vi "GetSyncRefnums.vi"(8 "error in (no error)":errorcluster, 11 "ModuleAdmin":refnum<class "ModuleAdmin.lvclass">) -> (0 "error out":errorcluster, 1 "rndzv_ModuleSync":T1, 2 "rndzv_EventSync":T1, 3 "rndzv_StopSync":T1)   [LabVIEW 2018, in "ModuleAdmin.lvlib" / "ModuleAdmin.lvclass"]
uses:
  ModuleAdmin.lvclass
  ModuleAdmin.lvclass/ModuleAdmin.ctl
  Accessors/Read CloneRegRef.vi
  CloneRegistration/CloneRegistration.lvclass
panel:
  out "new StopSync":bool
  out "new EventSync":bool
  out "new ModuleSync":bool
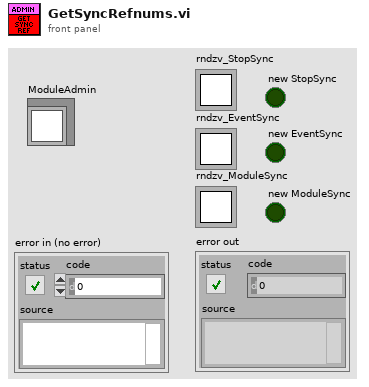
[diagram p1: front panel]
types:
  T1 = typedef "Rendezvous RefNum" = refnum<k1>
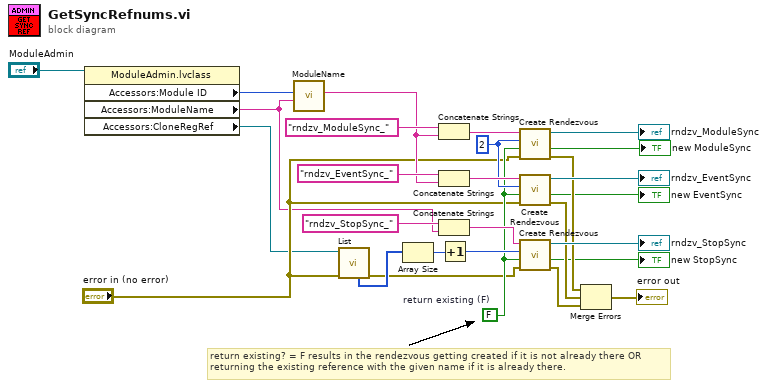
[diagram p0: block diagram]
diagram:
  w18 = 2 ("size (2)")
  w10 = FALSE  # return existing (F)
  # "return existing? = F results in the rendezvous getting created if it is not already there OR\nreturning the existing reference with the given name if it is already there."
  n1 = property class="ModuleAdmin.lvclass"(reference="ModuleAdmin") -> ("Accessors:Module ID"=w3:i32, "Accessors:ModuleName"=w1:string, "Accessors:CloneRegRef"=w2:refnum<data-value>)  [unwired: 1 in, 2 out]
  n2 = call "ModuleName.vi"("Name"=w1, "ModuleID"=w3) -> ("ModuleName"=w22:string)  [unwired: 9 in]
  n3 = call "List.vi"("error in (no error)"="error in (no error)", "CloneRegRef"=w2) -> ("error out"=w5:errorcluster, "Module IDs"=w28:i32[])  [unwired: 4 in, 4 out]
  n4 = Array Size(array=w28) -> (size(s)=w27:i32)
  n5 = Concatenate Strings("rndzv_ModuleSync_" ("string"), w22) -> (w21:string)
  n6 = Concatenate Strings("rndzv_EventSync_" ("string"), w22) -> (w20:string)
  n7 = Concatenate Strings("rndzv_StopSync_" ("string"), w1) -> (w19:string)
  n8 = Increment(x=w27) -> (x+1=w26:i32)
  n9 = call <vilib>:"Create Rendezvous.vi"("error in (no error)"="error in (no error)", "return existing (F)"=w10, "size (2)"=w18, "name (unnamed)"=w21) -> ("error out"=w13:errorcluster, "created new"=→"new ModuleSync":bool, "rendezvous"=→"rndzv_ModuleSync":T1)  [unwired: 1 in]
  n10 = call <vilib>:"Create Rendezvous.vi"("error in (no error)"="error in (no error)", "return existing (F)"=w10, "size (2)"=w18, "name (unnamed)"=w20) -> ("error out"=w14:errorcluster, "created new"=→"new EventSync":bool, "rendezvous"=→"rndzv_EventSync":T1)  [unwired: 1 in]
  n11 = call <vilib>:"Create Rendezvous.vi"("error in (no error)"=w5, "return existing (F)"=w10, "size (2)"=w26, "name (unnamed)"=w19) -> ("error out"=w12:errorcluster, "created new"=→"new StopSync":bool, "rendezvous"=→"rndzv_StopSync":T1)  [unwired: 1 in]
  n12 = Merge Errors(w13, w14, w12) -> (→"error out":errorcluster)
